vi "get_frame.vi"(8 "error in (no error)":errorcluster, 11 "DataFrame in":refnum<class "DataFrame.lvclass">) -> (0 "error out":errorcluster, 2 "dataframe":string, 3 "DataFrame out":refnum<class "DataFrame.lvclass">)   [LabVIEW 2017, in "DataFrame.lvclass"]
uses:
  DataFrame.lvclass
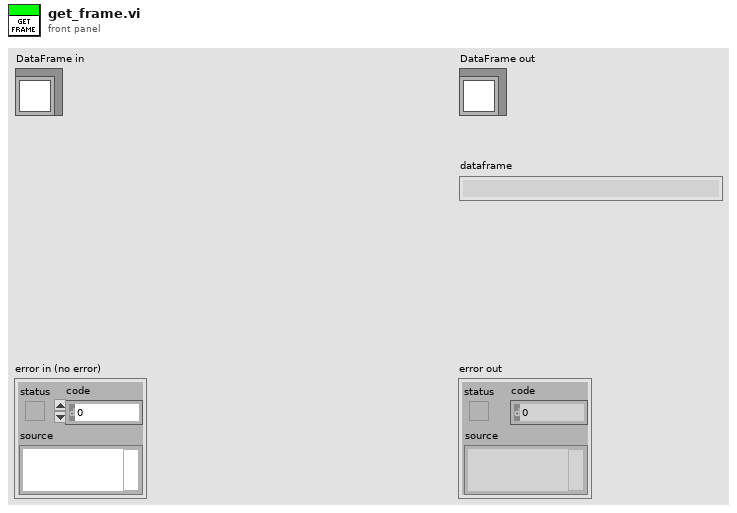
[diagram p1: front panel]
types:
  T1 = typedef "DataFrame.lvclass/command_type.ctl" = enum8{"read", "write", "blank_0", "blank_1", "blank_2", "blank_3", "blank_4", "blank_5", "blank_6", "blank_7", "blank_8", "blank_9", "blank_10", "blank_11", "blank_12", "exit", ""}
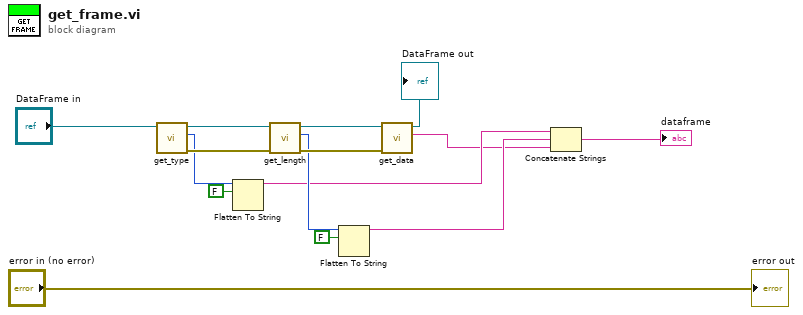
[diagram p0: block diagram]
diagram:
  n1 = call "get_type.vi"("DataFrame in"="DataFrame in") -> ("error out"=w14:errorcluster, "type"=w10:T1, "DataFrame out"=w12:refnum<class "DataFrame.lvclass">)  [unwired: 8 in]
  n2 = Flatten To String(anything=w10, prepend array or string size? (T)=FALSE) -> (data string=w6:string)  [unwired: 2 in, 2 out]
  n3 = call "get_length.vi"("error in (no error)"=w14, "DataFrame in"=w12) -> ("error out"=w13:errorcluster, "length"=w7:u32, "DataFrame out"=w11:refnum<class "DataFrame.lvclass">)  [unwired: 7 in]
  n4 = Flatten To String(anything=w7, prepend array or string size? (T)=FALSE) -> (data string=w5:string)  [unwired: 2 in, 2 out]
  n5 = call "get_data.vi"("error in (no error)"=w13, "DataFrame in"=w11) -> ("data"=w1:string, "DataFrame out"=→"DataFrame out":refnum<class "DataFrame.lvclass">)  [unwired: 7 in, 1 out]
  n6 = Concatenate Strings(w6, w5, w1) -> (→"dataframe":string)
  "error out" <- "error in (no error)"
